vi "Serial_Init.vi"(3 "error in (no error)":errorcluster) -> (0 "error out":errorcluster, 2 "VISA resource name out":refnum<visa-resource-name>)   [LabVIEW 2009, in "Serial.lvlib"]
doc: "Initializes serial port on compact RIO"
uses:
  Serial.lvlib
  <vilib>/Instr/_visa.llb/VISA Configure Serial Port (Instr).vi
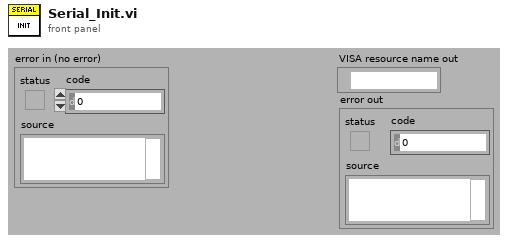
[diagram p1: front panel]
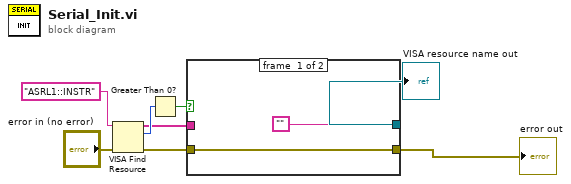
[diagram p0: block diagram]
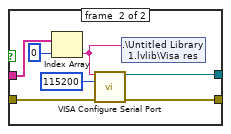
[diagram p2: hidden frame]
diagram:
  n1 = VISA Find Resource(8:"error in (no error)", 11:"ASRL1::INSTR" ("expression (\"?*\")")) -> (0:w3:errorcluster, 2:w7:u32, 3:w5:string[])  [unwired: 1 in]
  n2 = Greater Than 0?(x=w7) -> (x > 0?=w6:bool)
  n3 = case shown="True" w6 {
    tunnel: w5 -> [_ w17]
    tunnel: w3 -> [w10 w15]
    tunnel: ["" w12] -> w2
    tunnel: [w10 w14] -> w1
    frame #0 {
    }
    frame #1 {
      n4 = Index Array(array=w17, index=0) -> (element=w13:string)
      n5 = call-poly "VISA Configure Serial Port"("VISA resource name"=w13, "baud rate (9600)"=u32 115200, "error in (no error)"=w15) -> ("VISA resource name out"=w12:refnum<visa-resource-name>, "error out"=w14:errorcluster)  [unwired: 11 in]
      n6 = shared-variable ".\\Untitled Library 1.lvlib\\Visa res"(w13) -> ()  [unwired: 1 in, 1 out]
    }
  }
  "VISA resource name out" <- w2
  "error out" <- w1
